vi "EMTS_Simulator_2017_V1_Tansmitter_One_Plane_Multi_Orientation_KF_Test_CV-RobertTest.vi"() -> ()   [LabVIEW 2014]
uses:
  <vilib>/Utility/error.llb/DialogType.ctl
  <vilib>/Utility/file.llb/Write To Spreadsheet File (DBL).vi
  <vilib>/measure/NI_MAPro.lvlib
panel:
  out "Times":i32
  out "U_norm":dbl[](array[numeric])
  out "Time needed (s)":dbl format="%.2f"
  out "Signal Frequency":dbl=1000.0 format="%.2f"
  out "Numeric":i32=49
  in  "DC  (V)":dbl=1.0 format="%_3f"
  in  "Ramp Voltage (V)":dbl=1.0 format="%_3f"
  out "concatenated string":string="100*a*t"
  in  "Reset Signal":bool=TRUE
  in  "Sampling info (sine)":cluster{"Fs":dbl, "#s":dbl}={"Fs"=100000.0, "#s"=1001.0} {"Fs" format="%.2p"}
  in  "Sampling info (DC)":cluster{"Fs":dbl, "#s":dbl}={"Fs"=100000.0, "#s"=1000.0} {"Fs" format="%.2p"}
  in  "Theta_Guess":dbl=90.0
  in  "Phi_Guess":dbl=90.0
  in  "Z_Guess":dbl=0.05
  in  "Y_Guess":dbl
  in  "X_Guess":dbl
  out "Measured Voltage":dbl[][](graph)
  in  "Noise On ?":bool=TRUE
  out "delta_t":dbl=0.01001
  out "#s":dbl=1001.0
  in  "Select Waveform":u16(ring) items=["Sine Wave", "Ramp Wave", "DC Wave"]
  in  "Sampling info (ramp)":cluster{"Fs":dbl, "#s":dbl}={"Fs"=100000.0, "#s"=1000.0} {"Fs" format="%.2p"}
  in  "Sine Frequency (Hz)":dbl=1000.0 format="%.2f"
  in  "Sine Voltage (V)":dbl=1.0 format="%0.2p"
  out "Signal Generation":waveform(dbl)(graph)={"t0"=timestamp(0 s since 1904-01-01), "dt"=1e-05, "Y"=array[1001 elements]}
  in  "Noise Level (dBW)":dbl=-80.0
  in  "Sensor static ?":bool=TRUE
  in  "Reference length":sgl=4.0
  in  "Yaw 1 (deg)  4":dbl=90.0
  in  "Pitch 1 (deg) 4":dbl
  in  "Roll 1 (deg) 4":dbl
  in  "Yaw 1 (deg)  3":dbl
  in  "Pitch 1 (deg) 3":dbl
  in  "Roll 1 (deg) 3":dbl
  in  "Yaw 1 (deg)  2":dbl=90.0
  in  "Pitch 1 (deg) 2":dbl=90.0
  in  "Roll 1 (deg) 2":dbl
  in  "Reference Point":cluster{"X (m)":sgl, "Y (m)":sgl, "Z (m)":sgl}
  out "Real Yaw 8":dbl
  out "Real Pitch 8":dbl=90.0
  out "Real Yaw 7":dbl=5.0
  out "Real Pitch 7":dbl
  out "Real Yaw 6":dbl=240.0
  out "Real Pitch6":dbl=30.0
  out "Real Yaw 5":dbl=120.0
  out "Real Pitch 5":dbl=100.0
  out "Real Yaw 4":dbl=120.0
  out "Real Pitch 4":dbl=60.0
  out "Real Yaw 3":dbl=90.0
  out "Real Pitch 3":dbl=30.0
  out "Real Yaw 2":dbl=33.0
  out "Real Pitch 2":dbl=63.0
  out "Real Yaw 1":dbl=-85.0
  out "Real Pitch 1":dbl=92.0
  out "XYZ Coil8":cluster{dbl, dbl, dbl}={-0.04600000008940697, 0.0, 0.0}
  out "XYZ Coil7":cluster{dbl, dbl, dbl}={0.05000000074505806, 0.009999999776482582, 0.0}
  out "XYZ Coil6":cluster{dbl, dbl, dbl}={0.05000000074505806, 0.10000000149011612, 0.0}
  out "XYZ Coil5":cluster{dbl, dbl, dbl}={0.1550000011920929, 0.0, 0.0}
  out "XYZ Coil4":cluster{dbl, dbl, dbl}={0.05000000074505806, -0.10000000149011612, 0.0010000000474974513}
  out "XYZ Coil3":cluster{dbl, dbl, dbl}={-0.05000000074505806, -0.10000000149011612, 0.0}
  out "XYZ Coil2":cluster{dbl, dbl, dbl}={-0.14800000190734863, 0.003000000026077032, -0.0010000000474974513}
  out "XYZ Coil1":cluster{dbl, dbl, dbl}={-0.049000002443790436, 0.10500000417232513, -0.0020000000949949026}
  in  "DYaw8":dbl
  in  "DPitch8":dbl
  in  "DZ8":sgl
  in  "DY8":sgl
  in  "DX8":sgl=0.004
  in  "DYaw7":dbl=5.0
  in  "DPitch7":dbl
  in  "DZ7":sgl
  in  "DY7":sgl=0.01
  in  "DX7":sgl
  in  "DYaw6":dbl
  in  "DPitch6":dbl
  in  "DZ6":sgl
  in  "DY6":sgl
  in  "DX6":sgl
  in  "DYaw5":dbl
  in  "DPitch5":dbl=10.0
  in  "DZ5":sgl
  in  "DY5":sgl
  in  "DX5":sgl=0.005
  in  "DYaw4":dbl
  in  "DPitch4":dbl
  in  "DZ4":sgl=0.001
  in  "DY4":sgl
  in  "DX4":sgl
  in  "DYaw3":dbl
  in  "DPitch3":dbl
  in  "DZ3":sgl
  in  "DY3":sgl
  in  "DX3":sgl
  in  "DYaw2":dbl=3.0
  in  "DPitch2":dbl=3.0
  in  "DZ2":sgl=-0.001
  in  "DY2":sgl=0.003
  in  "DX2":sgl=0.002
  in  "DYaw1":dbl=5.0
  in  "DPitch1":dbl=2.0
  in  "DZ1":sgl=-0.002
  in  "DY1":sgl=0.005
  in  "DX1":sgl=0.001
  out "Yaw (deg)":dbl=45.0
  out "Pitch (deg)":dbl=45.0
  out "Sensor coil move":cluster{"X (m)":sgl, "Y (m)":sgl, "Z (m)":sgl}={"X (m)"=0.0, "Y (m)"=0.0, "Z (m)"=0.12}
  in  "stop":bool
  in  "Transmitters accurate ?":bool=TRUE
  out "Real sensor's P&O":dbl[](array[numeric])=[-0.25, -0.25, 0.05000000074505806, -180.0, -180.0] format="%_6g"
  out "Simulated voltage induced by each transmitter coil (V)":dbl[](array[numeric])=[-0.021471154535231914, -0.017236602261565384, -0.01016434944143931, -0.0024446696112596913, 0.011573940229747934, 0.026417718734482783, 0.025183921853267847, 0.015931276239022865]
  out "Estimated sensor's P&O":dbl[](array[numeric])=[-0.10001654341217367, -0.09996105359602137, 0.0500756336809607, -0.007269984859161761, 90.04621343342399] format="%.4f"
  in  "Radius of the sensor coil (m)":dbl=0.0002832
  in  "Radius of the transmitter coils (m)":dbl=0.015
  in  "Turns of the sensor coil":dbl=500.0
  in  "Length of the transmitter coils (m)":dbl=0.03
  in  "Turns of the transmitter coils":dbl=207.0
  in  "Pitch (deg)":dbl=45.0
  in  "Yaw (deg)":dbl=45.0
  in  "Roll (deg)":dbl
  in  "Sensor coil":cluster{"X (m)":sgl, "Y (m)":sgl, "Z (m)":sgl}={"X (m)"=0.0, "Y (m)"=0.0, "Z (m)"=0.12}
  in  "Pitch 8 (deg)":dbl=90.0
  in  "Yaw 8 (deg)":dbl
  in  "Roll 8 (deg)":dbl
  in  "Coil 8":cluster{"X (m)":sgl, "Y (m)":sgl, "Z (m)":sgl}={"X (m)"=-0.05, "Y (m)"=0.0, "Z (m)"=0.0}
  in  "Pitch 7 (deg)":dbl
  in  "Yaw 7 (deg)":dbl
  in  "Roll 7 (deg)":dbl
  in  "Coil 7":cluster{"X (m)":sgl, "Y (m)":sgl, "Z (m)":sgl}={"X (m)"=0.05, "Y (m)"=0.0, "Z (m)"=0.0}
  in  "Pitch 6 (deg)":dbl=30.0
  in  "Yaw 6 (deg)":dbl=240.0
  in  "Roll 6 (deg)":dbl
  in  "Coil 6":cluster{"X (m)":sgl, "Y (m)":sgl, "Z (m)":sgl}={"X (m)"=0.05, "Y (m)"=0.1, "Z (m)"=0.0}
  in  "Pitch 5 (deg)":dbl=90.0
  in  "Yaw 5 (deg)":dbl=120.0
  in  "Roll 5 (deg)":dbl
  in  "Coil 5":cluster{"X (m)":sgl, "Y (m)":sgl, "Z (m)":sgl}={"X (m)"=0.15, "Y (m)"=0.0, "Z (m)"=0.0}
  in  "Pitch 4 (deg)":dbl=60.0
  in  "Yaw 4 (deg)":dbl=120.0
  in  "Roll 4 (deg)":dbl
  in  "Coil 4":cluster{"X (m)":sgl, "Y (m)":sgl, "Z (m)":sgl}={"X (m)"=0.05, "Y (m)"=-0.1, "Z (m)"=0.0}
  in  "Pitch 3 (deg)":dbl=30.0
  in  "Yaw 3 (deg)":dbl=90.0
  in  "Roll 3 (deg)":dbl
  in  "Coil 3":cluster{"X (m)":sgl, "Y (m)":sgl, "Z (m)":sgl}={"X (m)"=-0.05, "Y (m)"=-0.1, "Z (m)"=0.0}
  in  "Pitch 2 (deg)":dbl=60.0
  in  "Yaw 2 (deg)":dbl=30.0
  in  "Roll 2 (deg)":dbl
  in  "Coil 2":cluster{"X (m)":sgl, "Y (m)":sgl, "Z (m)":sgl}={"X (m)"=-0.15, "Y (m)"=0.0, "Z (m)"=0.0}
  in  "Coil 1":cluster{"X (m)":sgl, "Y (m)":sgl, "Z (m)":sgl}={"X (m)"=-0.05, "Y (m)"=0.1, "Z (m)"=0.0}
  in  "Pitch (deg)":dbl=90.0
  in  "Roll 1 (deg)":dbl
  in  "Yaw 1 (deg)":dbl=-90.0
  out "3D Picture":refnum<vi>(3d-picture)
  in  "path to JPEG file":path
  # "Simulation Tool for 8 Channel AC Electromagnetic tracking system developed in OvG University \n                                                                    Copy Right 2016 received @ OvGU"
  # "Manual control of transmitter coils' shift"
  # "Changing positions (m) and orientations (degree) of the transmitter coils"
  # "Set coil parameter"
  # "Set P&Os of transmitter coil array"
  # "Author: Mengfei Li\n mengfei.li@ovgu.de"
  # "X (m)"
  # "Y (m)"
  # "Set sensor's P&O"
  # "Z (m)"
  # "Phi (deg)"
  # "Theta (deg)"
  # "Real position and orientation of the transmitter coils"
  # "Signal Generation Panel"
  # "Visualization of transmitter coil array and sensor coil"
  # "Real positions (m) and orientations (degree) of the transmitter coils"
  # "Initial guess value for \nsensor pose estimation"
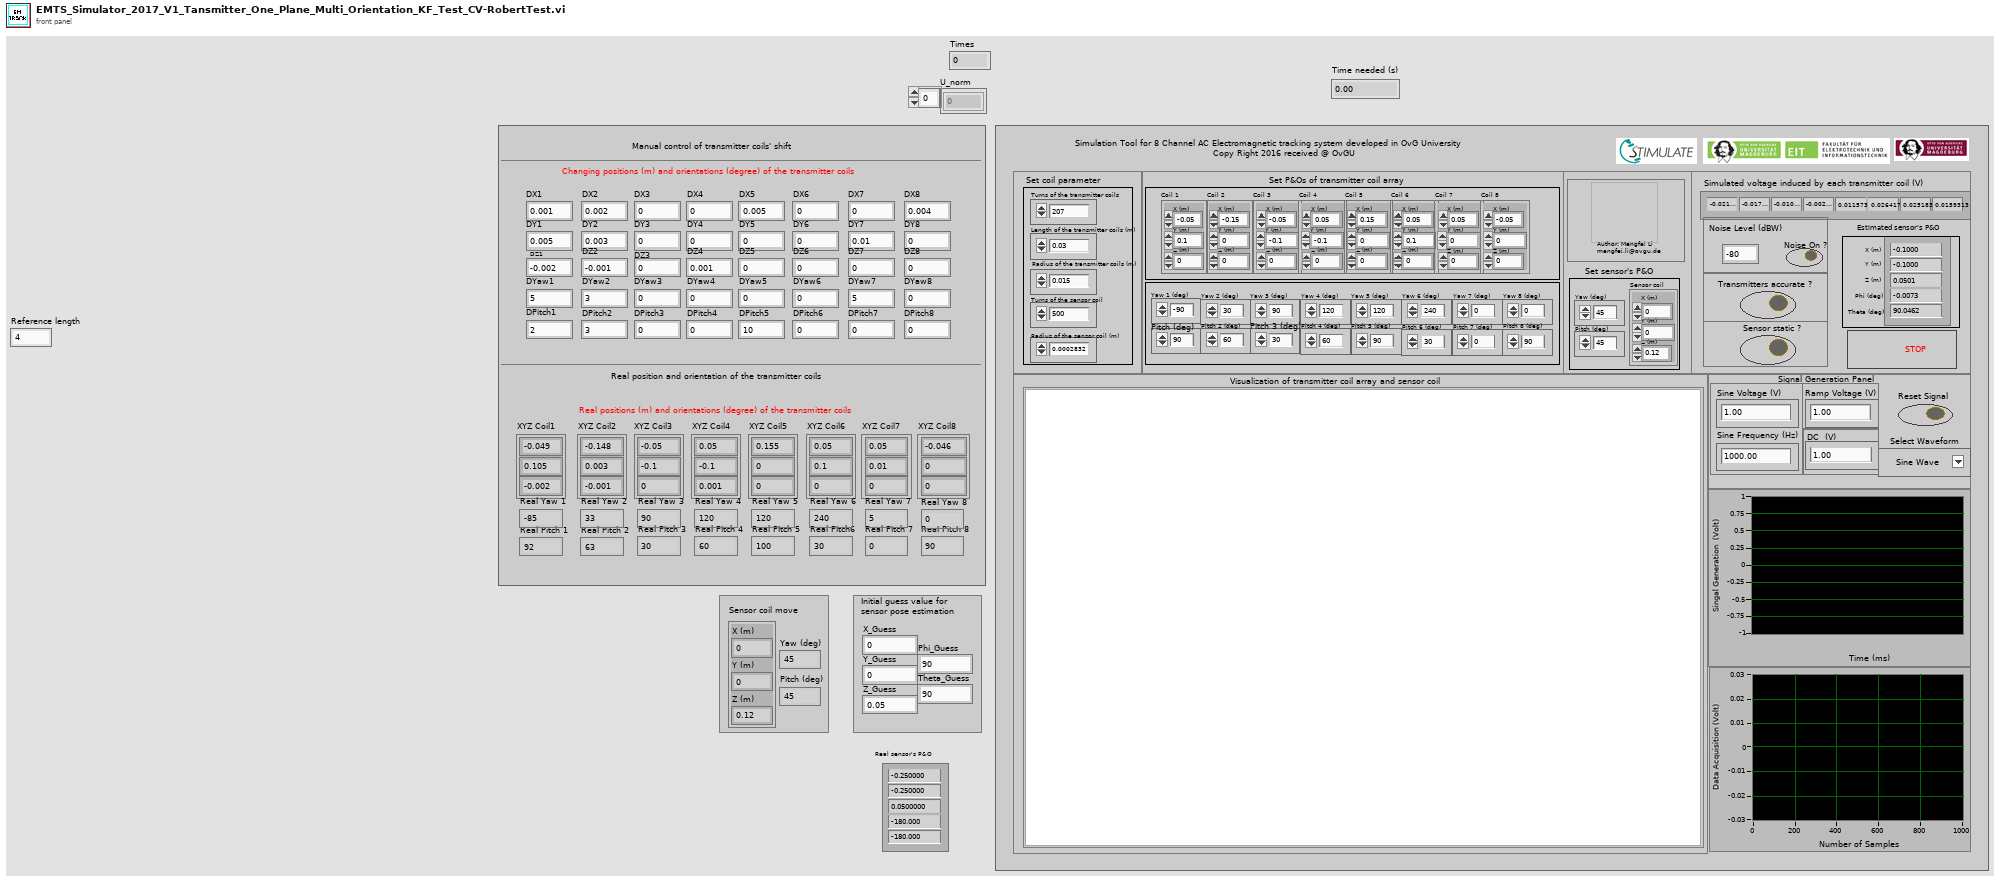
[diagram p1: front panel]
types:
  T1 = typedef "DialogType.ctl" = u16
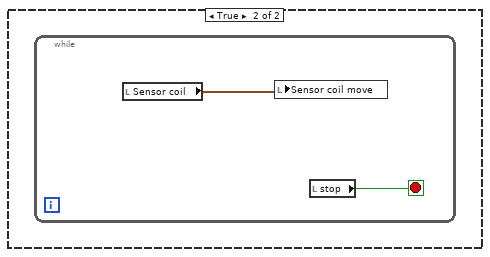
[diagram p2: hidden frame]
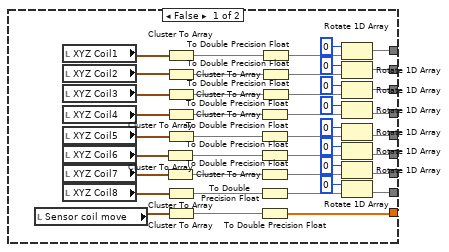
[diagram p4: hidden frame]
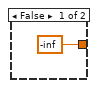
[diagram p5: hidden frame]
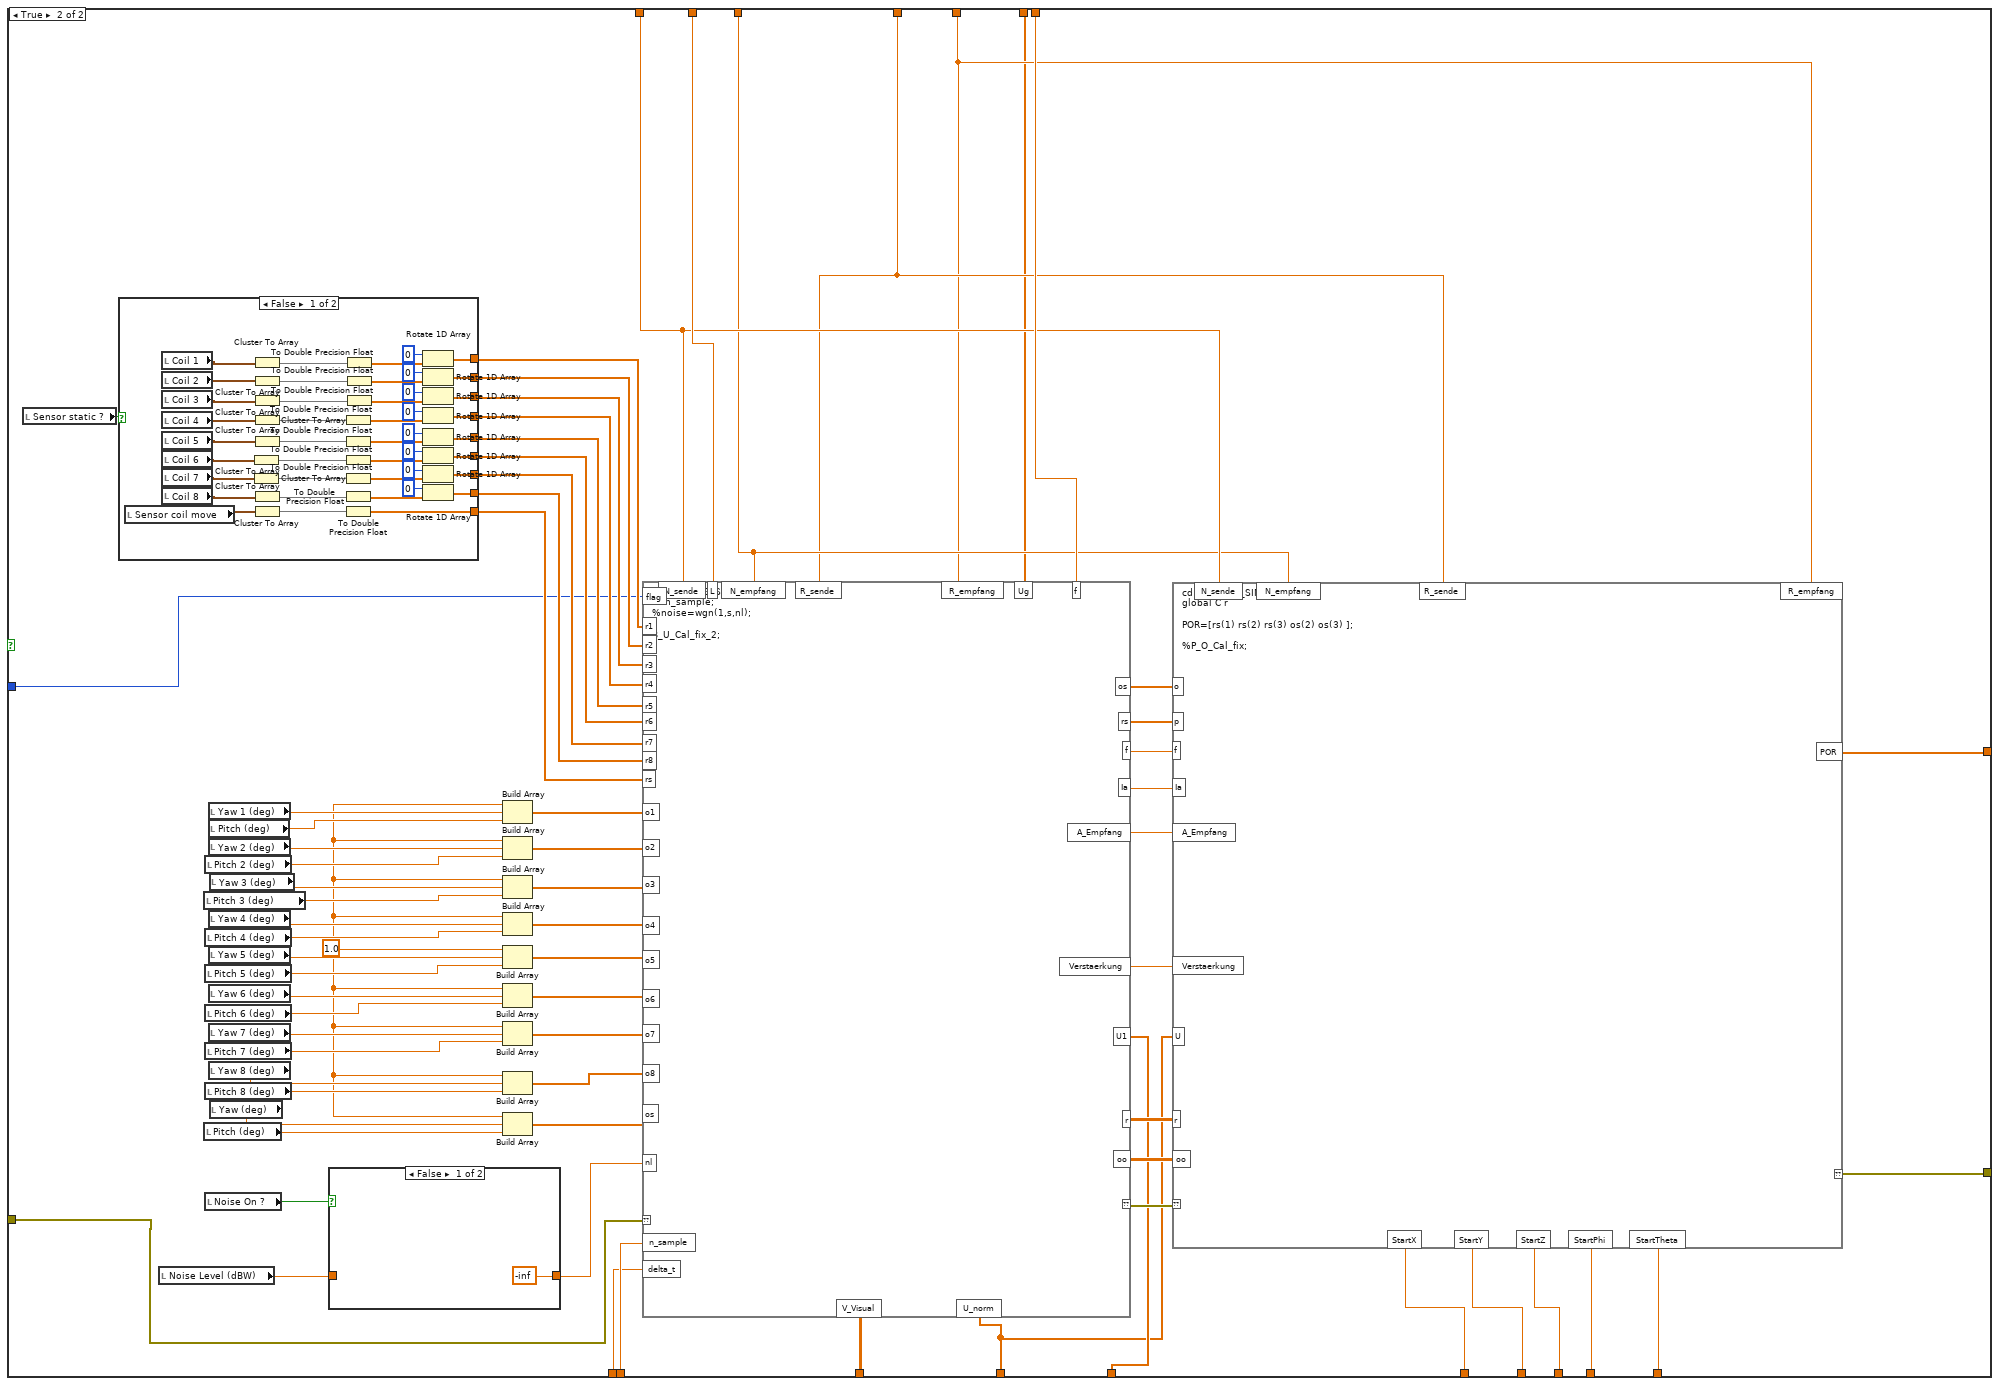
[diagram p6: hidden frame]
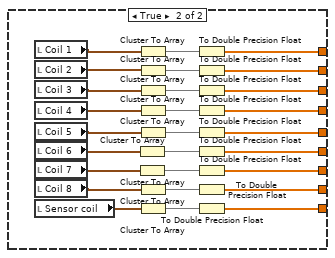
[diagram p7: hidden frame]
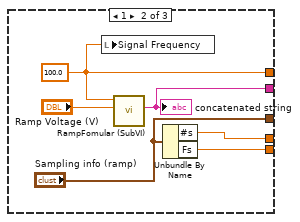
[diagram p12: hidden frame]
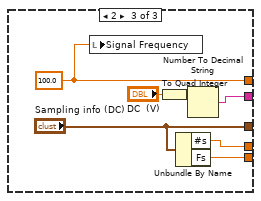
[diagram p13: hidden frame]
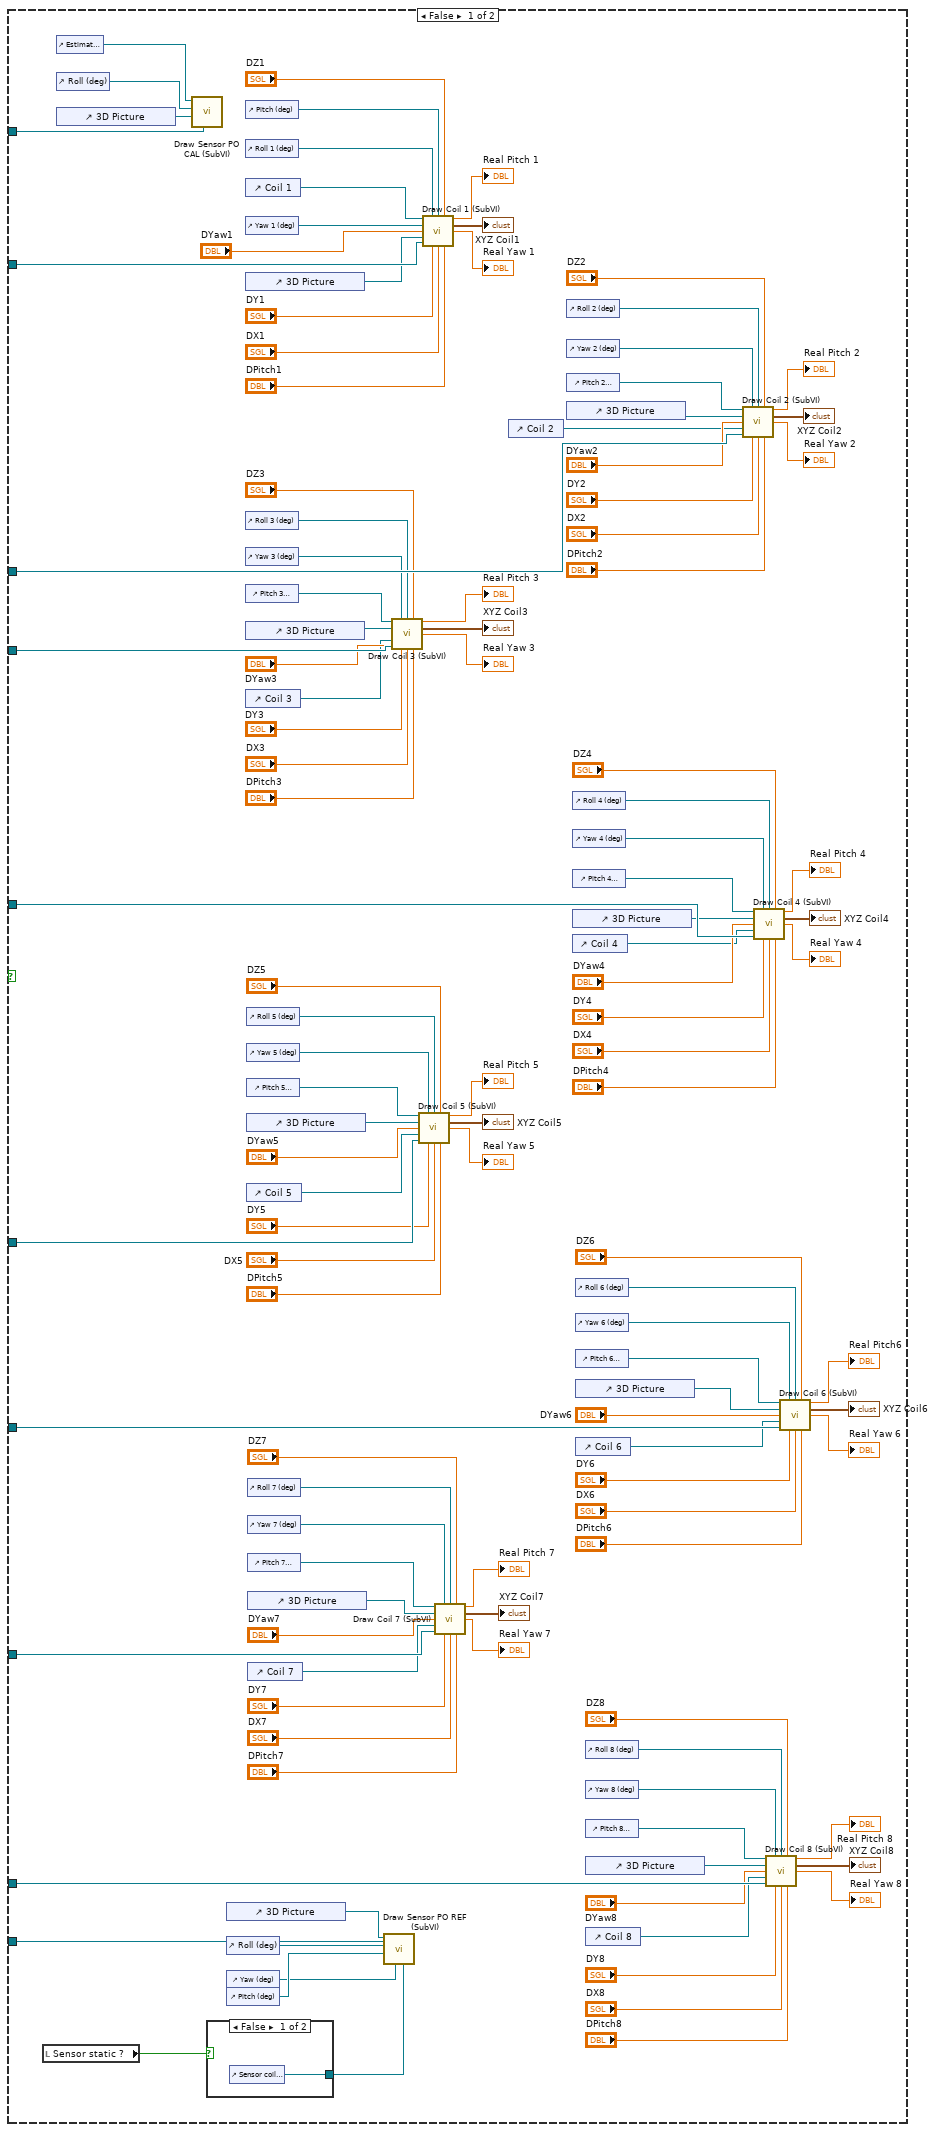
[diagram p14: hidden frame]
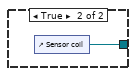
[diagram p15: hidden frame]
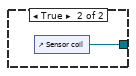
[diagram p16: hidden frame]
diagram:
  w7 = T1 3 items=["no dialog", "OK message", "continue or stop message", "OK message + warnings", "continue/stop + warnings"] ("type of dialog (OK msg:1)")
  # "This is an example here to move the sensor coil towards X, Y, Z axis. And this loop is where can be changed for testing the sensor movement models."
  # "Simulation of generated voltage"
  n1 = control-ref of="Length of the transmitter coils (m)"() -> (w15:refnum<vi>)
  n2 = control-ref of="Radius of the transmitter coils (m)"() -> (w16:refnum<vi>)
  n3 = call "Set Scenes (SubVI).vi"("Digital in"=w15, "path to JPEG file"="path to JPEG file", "reference"=w16) -> ("Scene:New Object"=w34:refnum<vi>, "Child 7"=w42:refnum<vi>, "SceneObject out"=w38:refnum<vi>, "Child"=w36:refnum<vi>, "Child 8"=w43:refnum<vi>, "Child 2"=w37:refnum<vi>, "Child 4"=w39:refnum<vi>, "Child 5"=w40:refnum<vi>, "Child 6"=w41:refnum<vi>)  [unwired: 4 in]
  n4 = control-ref of="Reference Point"() -> (w13:refnum<vi>)
  n5 = control-ref of="3D Picture"() -> (w14:refnum<vi>)
  n6 = while {
    stop <- w47 stop-if-true
    n7 = local read "Pitch (deg)"() -> (→"Pitch (deg)":dbl)
    n8 = local read "Yaw (deg)"() -> (→"Yaw (deg)":dbl)
    n9 = local read "stop"() -> (w47:bool)
    n10 = Wait (ms)(milliseconds to wait=u32 5) -> ()  [unwired: 1 out]
  }
  n11 = flat-sequence {
    tunnel: [w48] -> w5
    tunnel: w1 -> [w50]
    tunnel: w5 -> [w90]
    tunnel: [w89] -> w4
    frame #0 {
      n12 = Tick Count (ms)() -> (millisecond timer value=w48:u32)
      n13 = Wait (ms)(milliseconds to wait=u32 2000 ("millisecond timer value")) -> ()  [unwired: 1 out]
    }
    frame #1 {
      n14 = case shown="False" "Sensor static ?" {
        tunnel: w50 -> [w53 _]
        frame False {
          n15 = for {
            N: 100 -> [_]
            tunnel: w53 -> [w54]
            n16 = flat-sequence {
              tunnel: w54 -> [w72]
              frame #0 {
                n17 = local read "Sensor coil"() -> (w65:cluster{"X (m)":sgl, "Y (m)":sgl, "Z (m)":sgl})
                n18 = Unbundle(w65) -> ("X (m)"=w69:sgl, "Y (m)"=w56:sgl, "Z (m)"=w66:sgl)
                n19 = local read "Pitch (deg)"() -> (w59:dbl)
                n20 = Add(x=w69, y=sgl 0.001 ("x")) -> (x+y=w70:sgl)
                n21 = Add(x=sgl 0.0, y=w56) -> (x+y=w55:sgl)
                n22 = Add(x=sgl 0.0, y=w66) -> (x+y=w67:sgl)
                n23 = local read "Yaw (deg)"() -> (w62:dbl)
                n24 = Bundle(w70, w55, w67) -> (w64:cluster{sgl, sgl, sgl})  [unwired: 1 in]
                n25 = Add(x=w59, y=0.0) -> (x+y=w60:dbl)
                n26 = local write "Sensor coil move"(w64) -> ()
                n27 = local write "Sensor coil"(w64) -> ()
                n28 = local write "Pitch (deg)"(w60) -> ()
                n29 = Add(x=w62, y=0.0) -> (x+y=w61:dbl)
                n30 = local write "Yaw (deg)"(w61) -> ()
              }
              frame #1 {
                n31 = Set Occurrence(w72) -> ()
              }
              frame #2 {
                n32 = Wait (ms)(milliseconds to wait=u32 1200) -> ()  [unwired: 1 out]
              }
              frame #3 {
                n33 = local read "Simulated voltage induced by each transmitter coil (V)"() -> (w76:dbl[])
                n34 = local read "Real sensor's P&O"() -> (w74:dbl[])
                n35 = local read "U_norm"() -> (w75:dbl[])
                n36 = call-poly <vilib>:"Write To Spreadsheet File.vi"("format (%.3f)"="%.8f", "append to file? (new file:F)"=TRUE, "1D data"=w75, "file path (dialog if empty)"=path "d:/Um_Noise") -> ()  [unwired: 4 in, 1 out]
                n37 = call-poly <vilib>:"Write To Spreadsheet File.vi"("format (%.3f)"="%.8f", "append to file? (new file:F)"=TRUE, "1D data"=w74, "file path (dialog if empty)"=path "d:/POR") -> ()  [unwired: 4 in, 1 out]
                n38 = call-poly <vilib>:"Write To Spreadsheet File.vi"("format (%.3f)"="%.8f", "append to file? (new file:F)"=TRUE, "1D data"=w76, "file path (dialog if empty)"=path "d:/Um_NoNoise") -> ()  [unwired: 4 in, 1 out]
              }
              frame #4 {
                n39 = Wait (ms)(milliseconds to wait=u32 5) -> ()  [unwired: 1 out]
              }
            }
          }
        }
        frame True {
          n40 = while {
            stop <- w87 stop-if-true
            n41 = local read "Sensor coil"() -> (w88:cluster{"X (m)":sgl, "Y (m)":sgl, "Z (m)":sgl})
            n42 = local write "Sensor coil move"(w88) -> ()
            n43 = local read "stop"() -> (w87:bool)
          }
        }
      }
    }
    frame #2 {
      n44 = Tick Count (ms)() -> (millisecond timer value=w91:u32)
      n45 = Subtract(x=w91, y=w90) -> (x-y=w89:u32)
    }
  }
  n46 = call "Output Scenes (SubVI).vi"("SceneGraphDisplay in"=w14, "Yaw 1 (deg)  in"="Yaw 1 (deg)  2", "Roll 1 (deg) 3"="Roll 1 (deg) 3", "Roll 1 (deg) in"="Roll 1 (deg) 2", "Pitch 1 (deg) 3"="Pitch 1 (deg) 3", "Yaw 1 (deg)  4"="Yaw 1 (deg)  4", "Yaw 1 (deg)  3"="Yaw 1 (deg)  3", "Roll 1 (deg) 4"="Roll 1 (deg) 4", "Scene:New Object in"=w34, "Pitch 1 (deg) 4"="Pitch 1 (deg) 4", "reference"=w13, "Reference length"="Reference length", "Reference Point"="Reference Point", "Pitch 1 (deg) in"="Pitch 1 (deg) 2") -> ("SceneObject out"=w35:refnum<vi>, "Scene:New Object out"=w19:refnum<vi>, "Child"=w33:refnum<vi>)  [unwired: 3 in]
  n47 = while {
    tunnel: w43 -> [w103]
    tunnel: w42 -> [w104]
    tunnel: w41 -> [w102]
    tunnel: w40 -> [w101]
    tunnel: w39 -> [w100]
    tunnel: w38 -> [w99]
    tunnel: w37 -> [w98]
    tunnel: w36 -> [w97]
    tunnel: w35 -> [w96]
    tunnel: w33 -> [w95]
    tunnel: ["stop"] -> w30
    tunnel: w19 -> [w92]
    stop <- "stop" stop-if-true
    # "Loop 1: Coil Control and Visualization Loop"
    n48 = case shown="True" "Transmitters accurate ?" {
      tunnel: w104 -> [w227 w281]
      tunnel: w103 -> [w226 w280]
      tunnel: w102 -> [w225 w275]
      tunnel: w101 -> [w224 w270]
      tunnel: w100 -> [w223 w265]
      tunnel: w99 -> [w222 w260]
      tunnel: w98 -> [w221 w255]
      tunnel: w97 -> [w220 w250]
      tunnel: w96 -> [w219 w246]
      tunnel: w95 -> [w228 w245]
      frame False {
        n49 = local read "Sensor static ?"() -> (w107:bool)
        n50 = control-ref of="Estimated sensor's P&O"() -> (w177:refnum<vi>)
        n51 = control-ref of="Roll (deg)"() -> (w176:refnum<vi>)
        n52 = control-ref of="3D Picture"() -> (w175:refnum<vi>)
        n53 = call "Draw Sensor PO CAL (SubVI).vi"("Child"=w228, "SceneGraphDisp Refnum"=w175, "reference in"=w176, "Array in"=w177) -> ()  [unwired: 8 in]
        n54 = case shown="False" w107 {
          tunnel: [w229 w230] -> w106
          frame False {
            n55 = control-ref of="Sensor coil move"() -> (w229:refnum<vi>)
          }
          frame True {
            n56 = control-ref of="Sensor coil"() -> (w230:refnum<vi>)
          }
        }
        n57 = control-ref of="3D Picture"() -> (w108:refnum<vi>)
        n58 = control-ref of="Roll (deg)"() -> (w111:refnum<vi>)
        n59 = control-ref of="Yaw (deg)"() -> (w109:refnum<vi>)
        n60 = control-ref of="Pitch (deg)"() -> (w110:refnum<vi>)
        n61 = control-ref of="Pitch (deg)"() -> (w173:refnum<vi>)
        n62 = control-ref of="Roll 1 (deg)"() -> (w172:refnum<vi>)
        n63 = control-ref of="Coil 1"() -> (w174:refnum<vi>)
        n64 = control-ref of="Yaw 1 (deg)"() -> (w171:refnum<vi>)
        n65 = control-ref of="3D Picture"() -> (w170:refnum<vi>)
        n66 = control-ref of="Roll 3 (deg)"() -> (w158:refnum<vi>)
        n67 = control-ref of="Yaw 3 (deg)"() -> (w157:refnum<vi>)
        n68 = control-ref of="Pitch 3 (deg)"() -> (w159:refnum<vi>)
        n69 = control-ref of="3D Picture"() -> (w156:refnum<vi>)
        n70 = control-ref of="Coil 3"() -> (w155:refnum<vi>)
        n71 = control-ref of="Roll 5 (deg)"() -> (w142:refnum<vi>)
        n72 = control-ref of="Yaw 5 (deg)"() -> (w141:refnum<vi>)
        n73 = control-ref of="Pitch 5 (deg)"() -> (w143:refnum<vi>)
        n74 = control-ref of="3D Picture"() -> (w140:refnum<vi>)
        n75 = control-ref of="Coil 5"() -> (w139:refnum<vi>)
        n76 = control-ref of="Roll 7 (deg)"() -> (w126:refnum<vi>)
        n77 = control-ref of="Yaw 7 (deg)"() -> (w125:refnum<vi>)
        n78 = control-ref of="Pitch 7 (deg)"() -> (w127:refnum<vi>)
        n79 = control-ref of="3D Picture"() -> (w124:refnum<vi>)
        n80 = control-ref of="Coil 7"() -> (w123:refnum<vi>)
        n81 = call "Draw Sensor PO REF (SubVI).vi"("reference 4"=w106, "reference 3"=w109, "SceneObject in"=w219, "reference 2"=w110, "reference"=w111, "SceneGraphDisplay in"=w108) -> ()  [unwired: 6 in]
        n82 = call "Draw Coil 3 (SubVI).vi"("Digital in"=w159, "reference 3"=w157, "reference in"=w158, "DZ3"="DZ3", "SceneGraphDisp Refnum"=w156, "DPitch3"="DYaw3", "reference 4"=w155, "Child 6"=w225, "DY3"="DY3", "DX3"="DX3", "DYaw3"="DPitch3") -> ("Real Yaw 3"=→"Real Pitch 3":dbl, "XYZ Coil3"=→"XYZ Coil3":cluster{dbl, dbl, dbl}, "Real Pitch 3"=→"Real Yaw 3":dbl)  [unwired: 2 in]
        n83 = call "Draw Coil 5 (SubVI).vi"("Digital in"=w143, "reference 3"=w141, "reference in"=w142, "DZ5"="DZ5", "SceneGraphDisp Refnum"=w140, "DPitch5"="DYaw5", "reference 4"=w139, "Child 4"=w223, "DY5"="DY5", "DX5"="DX5", "DYaw5"="DPitch5") -> ("Real Yaw 5"=→"Real Pitch 5":dbl, "XYZ Coil5"=→"XYZ Coil5":cluster{dbl, dbl, dbl}, "Real Pitch 5"=→"Real Yaw 5":dbl)  [unwired: 2 in]
        n84 = call "Draw Coil 1 (SubVI).vi"("Cluster in"=w174, "reference 3"=w172, "reference in"=w173, "DZ1"="DZ1", "reference 4"=w171, "DPitch1"="DYaw1", "SceneGraphDisp Refnum"=w170, "Child 7"=w227, "DY1"="DY1", "DX1"="DX1", "DYaw1"="DPitch1") -> ("Real Yaw 1"=→"Real Pitch 1":dbl, "XYZ Coil1"=→"XYZ Coil1":cluster{dbl, dbl, dbl}, "Real Pitch 1"=→"Real Yaw 1":dbl)  [unwired: 2 in]
        n85 = call "Draw Coil 7 (SubVI).vi"("Digital in"=w127, "reference 3"=w125, "reference in"=w126, "DZ7"="DZ7", "SceneGraphDisp Refnum"=w124, "DPitch7"="DYaw7", "reference 4"=w123, "Child in"=w221, "DY7"="DY7", "DX7"="DX7", "DYaw7"="DPitch7") -> ("Real Yaw 7"=→"Real Pitch 7":dbl, "XYZ Coil7"=→"XYZ Coil7":cluster{dbl, dbl, dbl}, "Real Pitch 7"=→"Real Yaw 7":dbl)  [unwired: 2 in]
        n86 = control-ref of="Coil 2"() -> (w162:refnum<vi>)
        n87 = control-ref of="Roll 2 (deg)"() -> (w165:refnum<vi>)
        n88 = control-ref of="Yaw 2 (deg)"() -> (w164:refnum<vi>)
        n89 = control-ref of="Pitch 2 (deg)"() -> (w166:refnum<vi>)
        n90 = control-ref of="3D Picture"() -> (w163:refnum<vi>)
        n91 = control-ref of="Roll 4 (deg)"() -> (w150:refnum<vi>)
        n92 = control-ref of="Yaw 4 (deg)"() -> (w149:refnum<vi>)
        n93 = control-ref of="Pitch 4 (deg)"() -> (w151:refnum<vi>)
        n94 = control-ref of="3D Picture"() -> (w148:refnum<vi>)
        n95 = control-ref of="Coil 4"() -> (w147:refnum<vi>)
        n96 = control-ref of="Roll 6 (deg)"() -> (w134:refnum<vi>)
        n97 = control-ref of="Yaw 6 (deg)"() -> (w133:refnum<vi>)
        n98 = control-ref of="Pitch 6 (deg)"() -> (w135:refnum<vi>)
        n99 = control-ref of="3D Picture"() -> (w132:refnum<vi>)
        n100 = control-ref of="Coil 6"() -> (w131:refnum<vi>)
        n101 = control-ref of="Roll 8 (deg)"() -> (w118:refnum<vi>)
        n102 = control-ref of="Yaw 8 (deg)"() -> (w117:refnum<vi>)
        n103 = control-ref of="Pitch 8 (deg)"() -> (w119:refnum<vi>)
        n104 = control-ref of="3D Picture"() -> (w116:refnum<vi>)
        n105 = control-ref of="Coil 8"() -> (w115:refnum<vi>)
        n106 = call "Draw Coil 2 (SubVI).vi"("Digital in"=w166, "reference 3"=w164, "reference in"=w165, "DZ2"="DZ2", "SceneGraphDisp Refnum"=w163, "DPitch2"="DYaw2", "reference 4"=w162, "Child 8"=w226, "DY2"="DY2", "DX2"="DX2", "DYaw2"="DPitch2") -> ("Real Yaw 2"=→"Real Pitch 2":dbl, "XYZ Coil2"=→"XYZ Coil2":cluster{dbl, dbl, dbl}, "Numeric"=→"Real Yaw 2":dbl)  [unwired: 2 in]
        n107 = call "Draw Coil 4 (SubVI).vi"("Digital in"=w151, "reference 3"=w149, "reference in"=w150, "DZ4"="DZ4", "SceneGraphDisp Refnum"=w148, "DPitch4"="DYaw4", "reference 4"=w147, "Child 5"=w224, "DY4"="DY4", "DX4"="DX4", "DYaw4"="DPitch4") -> ("Real Yaw 4"=→"Real Pitch 4":dbl, "XYZ Coil4"=→"XYZ Coil4":cluster{dbl, dbl, dbl}, "Real Pitch 4"=→"Real Yaw 4":dbl)  [unwired: 2 in]
        n108 = call "Draw Coil 8 (SubVI).vi"("Digital in"=w119, "reference 3"=w117, "reference in"=w118, "DZ8"="DZ8", "SceneGraphDisp Refnum"=w116, "DPitch8"="DYaw8", "reference 4"=w115, "Child"=w220, "DY8"="DY8", "DX8"="DX8", "DYaw8"="DPitch8") -> ("Real Yaw 8"=→"Real Pitch 8":dbl, "XYZ Coil8"=→"XYZ Coil8":cluster{dbl, dbl, dbl}, "Real Pitch 8"=→"Real Yaw 8":dbl)  [unwired: 2 in]
        n109 = call "Draw Coil 6 (SubVI).vi"("Digital in"=w135, "reference 3"=w133, "reference in"=w134, "DZ6"="DZ6", "SceneGraphDisp Refnum"=w132, "DPitch6"="DYaw6", "reference 4"=w131, "SceneObject in"=w222, "DY6"="DY6", "DX6"="DX6", "DYaw6"="DPitch6") -> ("Real Yaw 6"=→"Real Pitch6":dbl, "XYZ Coil6"=→"XYZ Coil6":cluster{dbl, dbl, dbl}, "Real Pitch 6"=→"Real Yaw 6":dbl)  [unwired: 2 in]
      }
      frame True {
        n110 = control-ref of="3D Picture"() -> (w240:refnum<vi>)
        n111 = control-ref of="3D Picture"() -> (w238:refnum<vi>)
        n112 = control-ref of="3D Picture"() -> (w244:refnum<vi>)
        n113 = control-ref of="Estimated sensor's P&O"() -> (w243:refnum<vi>)
        n114 = control-ref of="Roll (deg)"() -> (w242:refnum<vi>)
        n115 = control-ref of="3D Picture"() -> (w236:refnum<vi>)
        n116 = control-ref of="3D Picture"() -> (w234:refnum<vi>)
        n117 = local read "Sensor static ?"() -> (w232:bool)
        n118 = call "Draw Coil 2_1 (SubVI).vi"("Roll 2 (deg)"="Roll 2 (deg)", "Yaw 2 (deg)"="Pitch 2 (deg)", "Pitch 2 (deg)"="Yaw 2 (deg)", "Child 8"=w280, "Coil in"="Coil 2", "SceneGraphDisplay in"=w240) -> ()  [unwired: 6 in]
        n119 = call "Draw Sensor PO CAL_1 (SubVI).vi"("Child"=w245, "reference 2"=w242, "reference"=w243, "SceneGraphDisplay in"=w244) -> ()  [unwired: 8 in]
        n120 = call "Draw Coil 4_1 (SubVI).vi"("Roll 4 (deg)"="Roll 4 (deg)", "Yaw 4 (deg)"="Pitch 4 (deg)", "Pitch 4 (deg)"="Yaw 4 (deg)", "SceneGraphDisp Refnum"=w238, "Coil 4"="Coil 4", "SceneObject in"=w270) -> ()  [unwired: 6 in]
        n121 = call "Draw Coil 6_1 (SubVI).vi"("Roll 6 (deg)"="Roll 6 (deg)", "Yaw 6 (deg)"="Pitch 6 (deg)", "Pitch 6 (deg)"="Yaw 6 (deg)", "SceneObject in"=w260, "Coil 6"="Coil 6", "SceneGraphDisplay in"=w236) -> ()  [unwired: 6 in]
        n122 = call "Draw Coil 8_1 (SubVI).vi"("Roll 8 (deg)"="Roll 8 (deg)", "Yaw 8 (deg)"="Pitch 8 (deg)", "Pitch 8 (deg)"="Yaw 8 (deg)", "Child"=w250, "Coil 8"="Coil 8", "SceneGraphDisplay in"=w234) -> ()  [unwired: 6 in]
        n123 = case shown="False" w232 {
          tunnel: [w290 w291] -> w231
          frame False {
            n124 = control-ref of="Sensor coil move"() -> (w290:refnum<vi>)
          }
          frame True {
            n125 = control-ref of="Sensor coil"() -> (w291:refnum<vi>)
          }
        }
        n126 = control-ref of="3D Picture"() -> (w237:refnum<vi>)
        n127 = control-ref of="3D Picture"() -> (w233:refnum<vi>)
        n128 = control-ref of="3D Picture"() -> (w235:refnum<vi>)
        n129 = control-ref of="3D Picture"() -> (w239:refnum<vi>)
        n130 = control-ref of="3D Picture"() -> (w241:refnum<vi>)
        n131 = call "Draw Coil 5_1 (SubVI).vi"("Roll 5 (deg)"="Roll 5 (deg)", "Yaw 5 (deg)"="Pitch 5 (deg)", "Pitch 5 (deg)"="Yaw 5 (deg)", "Child 4"=w265, "Coil 5"="Coil 5", "SceneGraphDisplay in"=w237) -> ()  [unwired: 6 in]
        n132 = call "Draw Coil 7_1 (SubVI).vi"("Roll 7 (deg)"="Roll 7 (deg)", "Yaw 7 (deg)"="Pitch 7 (deg)", "Pitch 7 (deg)"="Yaw 7 (deg)", "Child in"=w255, "Coil 7"="Coil 7", "SceneGraphDisplay in"=w235) -> ()  [unwired: 6 in]
        n133 = call "Draw Coil 3_1 (SubVI).vi"("Roll 3 (deg)"="Roll 3 (deg)", "Yaw 3 (deg)"="Pitch 3 (deg)", "Pitch 3 (deg)"="Yaw 3 (deg)", "SceneGraphDisp Refnum"=w239, "Coil 3"="Coil 3", "SceneObject in"=w275) -> ()  [unwired: 6 in]
        n134 = call "Draw Sensor PO REF_1 (SubVI).vi"("Roll (deg)"="Roll (deg)", "SceneObject in"=w246, "Pitch (deg)"="Yaw (deg)", "reference"=w231, "Yaw (deg)"="Pitch (deg)", "SceneGraphDisplay in"=w233) -> ()  [unwired: 6 in]
        n135 = call "Draw Coil 1_1 (SubVI).vi"("Roll 1 (deg)"="Roll 1 (deg)", "Yaw 1 (deg)"="Pitch (deg)", "Pitch 1 (deg)"="Yaw 1 (deg)", "Child 7"=w281, "Coil 1"="Coil 1", "SceneGraphDisplay in"=w241) -> ()  [unwired: 6 in]
      }
    }
    n136 = Wait (ms)(milliseconds to wait=u32 20) -> ()  [unwired: 1 out]
    "3D Picture" <- w92
  }
  n137 = local read "stop"() -> (w32:bool)
  n138 = Not Or(1:w32, 2:w30) -> (0:w31:bool)
  n139 = local write "stop"(w31) -> ()
  n140 = disable-structure shown="Disabled" {
    frame Disabled {
      n141 = flat-sequence {
        frame #0 {
          n142 = Wait (ms)(milliseconds to wait=u32 4000) -> ()  [unwired: 1 out]
        }
        frame #1 {
          n143 = for {
            N: 50 -> [_]
            shift-right: [w302] -> _
            shift-left: _ -> [_]
            shift-right: [w301] -> _
            shift-left: _ -> [w300]
            shift-left: _ -> [w294]
            shift-left: _ -> [w296]
            i -> [w305]
            n144 = Not Equal?(x=w300, y=w294) -> (x != y?=w299:bool[])
            n145 = Index Array(array=w299, index=0) -> (element=w297:bool)
            n146 = case shown="False" w297 {
              tunnel: [i32[] [0, 0, 0, 0, 0] w312] -> w295
              tunnel: w294 -> [_ w312]
              frame False {
              }
              frame True {
              }
            }
            n147 = Wait (ms)(milliseconds to wait=u32 500) -> ()  [unwired: 1 out]
            n148 = call-poly <vilib>:"Write To Spreadsheet File.vi"("format (%.3f)"="%.8f", "append to file? (new file:F)"=TRUE, "1D data"=w296, "file path (dialog if empty)"=path "d:/test2016/paper2/eval1/POE") -> ()  [unwired: 4 in, 1 out]
            n149 = local read "Estimated sensor's P&O"() -> (w302:dbl[])
            n150 = local read "Real sensor's P&O"() -> (w301:dbl[])
            n151 = call-poly <vilib>:"Write To Spreadsheet File.vi"("format (%.3f)"="%.8f", "append to file? (new file:F)"=TRUE, "1D data"=w295, "file path (dialog if empty)"=path "d:/test2016/paper2/eval1/POR") -> ()  [unwired: 4 in, 1 out]
            "Numeric" <- w305
          }
        }
      }
    }
    frame Enabled {
    }
  }
  n152 = Generate Occurrence() -> (w1:refnum<k4>)
  n153 = while {
    tunnel: [w319] -> w6
    tunnel: "X_Guess" -> [w318]
    tunnel: "Y_Guess" -> [w317]
    tunnel: "Z_Guess" -> [w316]
    tunnel: "Phi_Guess" -> [w315]
    tunnel: "Theta_Guess" -> [w314]
    tunnel: w1 -> [w313]
    stop <- w320 stop-if-true
    n154 = flat-sequence {
      tunnel: w313 -> [w321]
      tunnel: [w344] -> w320
      tunnel: [w336] -> w319
      tunnel: w318 -> [w327]
      tunnel: w317 -> [w326]
      tunnel: w316 -> [w325]
      tunnel: w315 -> [w324]
      tunnel: w314 -> [w323]
      frame #0 {
        n155 = Wait on Occurrence(2:w321) -> ()  [unwired: 2 in, 1 out]
      }
      frame #1 {
        n156 = local read "Transmitters accurate ?"() -> (w337:bool)
        n157 = local read "Select Waveform"() -> (w331:u16)
        n158 = local read "Signal Generation"() -> (w330:waveform(dbl))
        n159 = Unbundle By Name(w330) -> ("Y"=w329:dbl[])
        n160 = local read "#s"() -> (w333:dbl)
        n161 = local read "delta_t"() -> (w332:dbl)
        n162 = local read "Sine Frequency (Hz)"() -> (w334:dbl)
        n163 = case shown="False" w337 {
          tunnel: w334 -> [w422 w564]
          tunnel: "Length of the transmitter coils (m)" -> [w423 w563]
          tunnel: "Turns of the transmitter coils" -> [w419 w559]
          tunnel: "Turns of the sensor coil" -> [w418 w558]
          tunnel: "Radius of the transmitter coils (m)" -> [w417 w557]
          tunnel: "Radius of the sensor coil (m)" -> [w416 w556]
          tunnel: [w420 w533] -> w345
          tunnel: [w421 w551] -> w343
          tunnel: [w390 w548] -> w336
          tunnel: errorcluster {"status"=FALSE, "code"=0, "source"=""} ("error in") -> [w385 w532]
          tunnel: w333 -> [w389 w547]
          tunnel: w332 -> [w388 w546]
          tunnel: w331 -> [w387 w545]
          tunnel: w329 -> [w386 w544]
          tunnel: [w381 w540] -> w328
          tunnel: w327 -> [w379 w534]
          tunnel: w326 -> [w378 w539]
          tunnel: w325 -> [w377 w538]
          tunnel: w324 -> [w376 w537]
          tunnel: w323 -> [w375 w536]
          tunnel: [w347 w531] -> w322
          frame False {
            w374 = 1.0
            w442 = 1.0
            n164 = local read "Sensor static ?"() -> (w348:bool)
            n165 = case shown="True" w348 {
              tunnel: [w467 w508] -> w430
              tunnel: [w459 w516] -> w415
              tunnel: [w460 w515] -> w414
              tunnel: [w461 w514] -> w413
              tunnel: [w462 w513] -> w412
              tunnel: [w463 w512] -> w411
              tunnel: [w464 w511] -> w410
              tunnel: [w465 w510] -> w409
              tunnel: [w466 w509] -> w408
              frame False {
                n166 = local read "Sensor coil move"() -> (w468:cluster{"X (m)":sgl, "Y (m)":sgl, "Z (m)":sgl})
                n167 = local read "XYZ Coil1"() -> (w501:cluster{dbl, dbl, dbl})
                n168 = local read "XYZ Coil2"() -> (w500:cluster{dbl, dbl, dbl})
                n169 = local read "XYZ Coil3"() -> (w499:cluster{dbl, dbl, dbl})
                n170 = local read "XYZ Coil4"() -> (w498:cluster{dbl, dbl, dbl})
                n171 = local read "XYZ Coil5"() -> (w497:cluster{dbl, dbl, dbl})
                n172 = local read "XYZ Coil6"() -> (w496:cluster{dbl, dbl, dbl})
                n173 = local read "XYZ Coil7"() -> (w495:cluster{dbl, dbl, dbl})
                n174 = local read "XYZ Coil8"() -> (w494:cluster{dbl, dbl, dbl})
                n175 = Cluster To Array(cluster=w496) -> (array=w489:dbl[])
                n176 = Cluster To Array(cluster=w495) -> (array=w488:dbl[])
                n177 = Cluster To Array(cluster=w501) -> (array=w477:dbl[])
                n178 = Cluster To Array(cluster=w500) -> (array=w493:dbl[])
                n179 = Cluster To Array(cluster=w499) -> (array=w492:dbl[])
                n180 = Cluster To Array(cluster=w498) -> (array=w491:dbl[])
                n181 = Cluster To Array(cluster=w497) -> (array=w490:dbl[])
                n182 = Cluster To Array(cluster=w494) -> (array=w487:dbl[])
                n183 = Cluster To Array(cluster=w468) -> (array=w486:sgl[])
                n184 = To Double Precision Float(number=w491) -> (double precision float=w482:dbl[])
                n185 = To Double Precision Float(number=w490) -> (double precision float=w481:dbl[])
                n186 = To Double Precision Float(number=w489) -> (double precision float=w480:dbl[])
                n187 = To Double Precision Float(number=w488) -> (double precision float=w479:dbl[])
                n188 = To Double Precision Float(number=w487) -> (double precision float=w478:dbl[])
                n189 = To Double Precision Float(number=w486) -> (double precision float=w467:dbl[])
                n190 = To Double Precision Float(number=w477) -> (double precision float=w485:dbl[])
                n191 = To Double Precision Float(number=w493) -> (double precision float=w484:dbl[])
                n192 = To Double Precision Float(number=w492) -> (double precision float=w483:dbl[])
                n193 = Rotate 1D Array(1:w485, 2:0 ("n")) -> (0:w459:dbl[])
                n194 = Rotate 1D Array(1:w484, 2:0 ("n")) -> (0:w460:dbl[])
                n195 = Rotate 1D Array(1:w483, 2:0 ("n")) -> (0:w461:dbl[])
                n196 = Rotate 1D Array(1:w482, 2:0 ("n")) -> (0:w462:dbl[])
                n197 = Rotate 1D Array(1:w481, 2:0 ("n")) -> (0:w463:dbl[])
                n198 = Rotate 1D Array(1:w480, 2:0 ("n")) -> (0:w464:dbl[])
                n199 = Rotate 1D Array(1:w479, 2:0 ("n")) -> (0:w465:dbl[])
                n200 = Rotate 1D Array(1:w478, 2:0 ("n")) -> (0:w466:dbl[])
              }
              frame True {
                n201 = local read "XYZ Coil1"() -> (w528:cluster{dbl, dbl, dbl})
                n202 = local read "XYZ Coil2"() -> (w527:cluster{dbl, dbl, dbl})
                n203 = local read "XYZ Coil3"() -> (w507:cluster{dbl, dbl, dbl})
                n204 = local read "XYZ Coil4"() -> (w506:cluster{dbl, dbl, dbl})
                n205 = local read "XYZ Coil5"() -> (w505:cluster{dbl, dbl, dbl})
                n206 = local read "XYZ Coil6"() -> (w504:cluster{dbl, dbl, dbl})
                n207 = local read "XYZ Coil7"() -> (w503:cluster{dbl, dbl, dbl})
                n208 = local read "XYZ Coil8"() -> (w502:cluster{dbl, dbl, dbl})
                n209 = local read "Sensor coil"() -> (w526:cluster{"X (m)":sgl, "Y (m)":sgl, "Z (m)":sgl})
                n210 = Cluster To Array(cluster=w504) -> (array=w521:dbl[])
                n211 = Cluster To Array(cluster=w503) -> (array=w520:dbl[])
                n212 = Cluster To Array(cluster=w528) -> (array=w517:dbl[])
                n213 = Cluster To Array(cluster=w527) -> (array=w525:dbl[])
                n214 = Cluster To Array(cluster=w507) -> (array=w524:dbl[])
                n215 = Cluster To Array(cluster=w506) -> (array=w523:dbl[])
                n216 = Cluster To Array(cluster=w505) -> (array=w522:dbl[])
                n217 = Cluster To Array(cluster=w502) -> (array=w519:dbl[])
                n218 = Cluster To Array(cluster=w526) -> (array=w518:sgl[])
                n219 = To Double Precision Float(number=w517) -> (double precision float=w516:dbl[])
                n220 = To Double Precision Float(number=w525) -> (double precision float=w515:dbl[])
                n221 = To Double Precision Float(number=w524) -> (double precision float=w514:dbl[])
                n222 = To Double Precision Float(number=w523) -> (double precision float=w513:dbl[])
                n223 = To Double Precision Float(number=w522) -> (double precision float=w512:dbl[])
                n224 = To Double Precision Float(number=w521) -> (double precision float=w511:dbl[])
                n225 = To Double Precision Float(number=w520) -> (double precision float=w510:dbl[])
                n226 = To Double Precision Float(number=w519) -> (double precision float=w509:dbl[])
                n227 = To Double Precision Float(number=w518) -> (double precision float=w508:dbl[])
              }
            }
            n228 = local read "Real Pitch 1"() -> (w457:dbl)
            n229 = local read "Real Pitch 2"() -> (w455:dbl)
            n230 = local read "Real Pitch 3"() -> (w453:dbl)
            n231 = local read "Real Pitch 4"() -> (w451:dbl)
            n232 = local read "Real Pitch 5"() -> (w449:dbl)
            n233 = local read "Real Pitch 7"() -> (w445:dbl)
            n234 = local read "Real Pitch 8"() -> (w443:dbl)
            n235 = local read "Real Pitch6"() -> (w447:dbl)
            n236 = local read "Pitch (deg)"() -> (w441:dbl)
            n237 = local read "Yaw (deg)"() -> (w440:dbl)
            n238 = local read "Real Yaw 1"() -> (w458:dbl)
            n239 = local read "Real Yaw 2"() -> (w456:dbl)
            n240 = local read "Real Yaw 3"() -> (w454:dbl)
            n241 = local read "Real Yaw 4"() -> (w452:dbl)
            n242 = local read "Real Yaw 5"() -> (w450:dbl)
            n243 = local read "Real Yaw 6"() -> (w448:dbl)
            n244 = local read "Real Yaw 7"() -> (w446:dbl)
            n245 = local read "Real Yaw 8"() -> (w444:dbl)
            n246 = case shown="True" "Noise On ?" {
              tunnel: [-inf w530] -> w382
              tunnel: "Noise Level (dBW)" -> [_ w530]
              frame False {
              }
              frame True {
              }
            }
            n247 = Build Array(w442, w458, w457) -> (w439:dbl[])
            n248 = Build Array(w442, w456, w455) -> (w438:dbl[])
            n249 = Build Array(w442, w454, w453) -> (w437:dbl[])
            n250 = Build Array(w442, w452, w451) -> (w436:dbl[])
            n251 = Build Array(w442, w450, w449) -> (w435:dbl[])
            n252 = Build Array(w442, w448, w447) -> (w434:dbl[])
            n253 = Build Array(w442, w446, w445) -> (w433:dbl[])
            n254 = Build Array(w442, w444, w443) -> (w432:dbl[])
            n255 = Build Array(w442, w441, w440) -> (w431:dbl[])
            n256 = script code="cd ('C:\\EMTS_SIMU')\ns=n_sample;\n% noise=wgn(1,s,nl);\n\nB_U_Cal_fix_2;"("??"=w385, "r1"=w415, "r2"=w414, "r3"=w413, "r4"=w412, "r5"=w411, "r6"=w410, "r7"=w409, "r8"=w408, "rs"=w430, "o1"=w439, "o2"=w438, "o3"=w437, "o4"=w436, "o5"=w435, "o6"=w434, "o7"=w433, "o8"=w432, "os"=w431, "N_sende"=w419, "L"=w423, "N_empfang"=w418, "R_sende"=w417, "R_empfang"=w416, "Ug"=w386, "f"=w422, "nl"=w382, "n_sample"=w389, "delta_t"=w388, "flag"=w387) -> ("??"=w391:errorcluster, "rs"=w429:dbl[], "f"=w428:dbl, "os"=w427:dbl[], "Ia"=w426:dbl, "A_Empfang"=w425:dbl, "Verstaerkung"=w424:dbl, "U1"=w420:dbl[], "V_Visual"=w381:dbl[][], "U_norm"=w347:dbl[])
            n257 = local read "Pitch 3 (deg)"() -> (w363:dbl)
            n258 = local read "Pitch 2 (deg)"() -> (w361:dbl)
            n259 = local read "Pitch 4 (deg)"() -> (w365:dbl)
            n260 = local read "Pitch 5 (deg)"() -> (w367:dbl)
            n261 = local read "Pitch 6 (deg)"() -> (w369:dbl)
            n262 = local read "Pitch 7 (deg)"() -> (w371:dbl)
            n263 = local read "Pitch 8 (deg)"() -> (w373:dbl)
            n264 = local read "Yaw 1 (deg)"() -> (w358:dbl)
            n265 = local read "Pitch (deg)"() -> (w359:dbl)
            n266 = local read "Yaw 2 (deg)"() -> (w360:dbl)
            n267 = local read "Yaw 4 (deg)"() -> (w364:dbl)
            n268 = local read "Yaw 5 (deg)"() -> (w366:dbl)
            n269 = local read "Yaw 6 (deg)"() -> (w368:dbl)
            n270 = local read "Yaw 7 (deg)"() -> (w370:dbl)
            n271 = local read "Yaw 8 (deg)"() -> (w372:dbl)
            n272 = local read "Yaw 3 (deg)"() -> (w362:dbl)
            n273 = local read "Coil 1"() -> (w407:cluster{"X (m)":sgl, "Y (m)":sgl, "Z (m)":sgl})
            n274 = local read "Coil 2"() -> (w406:cluster{"X (m)":sgl, "Y (m)":sgl, "Z (m)":sgl})
            n275 = local read "Coil 3"() -> (w405:cluster{"X (m)":sgl, "Y (m)":sgl, "Z (m)":sgl})
            n276 = local read "Coil 4"() -> (w404:cluster{"X (m)":sgl, "Y (m)":sgl, "Z (m)":sgl})
            n277 = local read "Coil 5"() -> (w403:cluster{"X (m)":sgl, "Y (m)":sgl, "Z (m)":sgl})
            n278 = local read "Coil 6"() -> (w402:cluster{"X (m)":sgl, "Y (m)":sgl, "Z (m)":sgl})
            n279 = local read "Coil 7"() -> (w401:cluster{"X (m)":sgl, "Y (m)":sgl, "Z (m)":sgl})
            n280 = local read "Coil 8"() -> (w400:cluster{"X (m)":sgl, "Y (m)":sgl, "Z (m)":sgl})
            n281 = Cluster To Array(cluster=w407) -> (array=w399:sgl[])
            n282 = Cluster To Array(cluster=w406) -> (array=w398:sgl[])
            n283 = Cluster To Array(cluster=w405) -> (array=w397:sgl[])
            n284 = Cluster To Array(cluster=w404) -> (array=w396:sgl[])
            n285 = Cluster To Array(cluster=w403) -> (array=w395:sgl[])
            n286 = Cluster To Array(cluster=w402) -> (array=w394:sgl[])
            n287 = Cluster To Array(cluster=w401) -> (array=w393:sgl[])
            n288 = Cluster To Array(cluster=w400) -> (array=w392:sgl[])
            n289 = Build Array(w399, w398, w397, w396, w395, w394, w393, w392) -> (w380:sgl[][])
            n290 = Build Array(w374, w358, w359) -> (w357:dbl[])
            n291 = Build Array(w374, w360, w361) -> (w356:dbl[])
            n292 = Build Array(w374, w362, w363) -> (w355:dbl[])
            n293 = Build Array(w374, w364, w365) -> (w354:dbl[])
            n294 = Build Array(w374, w366, w367) -> (w353:dbl[])
            n295 = Build Array(w374, w368, w369) -> (w352:dbl[])
            n296 = Build Array(w374, w370, w371) -> (w351:dbl[])
            n297 = Build Array(w374, w372, w373) -> (w350:dbl[])
            n298 = Build Array(w357, w356, w355, w354, w353, w352, w351, w350) -> (w349:dbl[][])
            n299 = script code="cd ('C:\\EMTS_SIMU')\nglobal C r \n\n\nPOR=[rs(1) rs(2) rs(3) os(2) os(3) ];\n\n%P_O_Cal_fix;"("??"=w391, "p"=w429, "f"=w428, "o"=w427, "N_sende"=w419, "N_empfang"=w418, "R_sende"=w417, "R_empfang"=w416, "Ia"=w426, "A_Empfang"=w425, "Verstaerkung"=w424, "U"=w347, "r"=w380, "StartX"=w379, "StartY"=w378, "StartZ"=w377, "StartPhi"=w376, "StartTheta"=w375, "oo"=w349) -> ("??"=w390:errorcluster, "POR"=w421:dbl[])
          }
          frame True {
            w585 = 1.0
            n300 = local read "Sensor static ?"() -> (w535:bool)
            n301 = case shown="False" w535 {
              tunnel: [w610 w654] -> w581
              tunnel: [w609 w653] -> w572
              tunnel: [w608 w652] -> w571
              tunnel: [w607 w651] -> w570
              tunnel: [w606 w650] -> w569
              tunnel: [w605 w649] -> w568
              tunnel: [w604 w648] -> w567
              tunnel: [w603 w647] -> w566
              tunnel: [w602 w646] -> w565
              frame False {
                n302 = local read "Sensor coil move"() -> (w611:cluster{"X (m)":sgl, "Y (m)":sgl, "Z (m)":sgl})
                n303 = local read "Coil 1"() -> (w644:cluster{"X (m)":sgl, "Y (m)":sgl, "Z (m)":sgl})
                n304 = local read "Coil 2"() -> (w643:cluster{"X (m)":sgl, "Y (m)":sgl, "Z (m)":sgl})
                n305 = local read "Coil 3"() -> (w642:cluster{"X (m)":sgl, "Y (m)":sgl, "Z (m)":sgl})
                n306 = local read "Coil 4"() -> (w641:cluster{"X (m)":sgl, "Y (m)":sgl, "Z (m)":sgl})
                n307 = local read "Coil 5"() -> (w640:cluster{"X (m)":sgl, "Y (m)":sgl, "Z (m)":sgl})
                n308 = local read "Coil 6"() -> (w639:cluster{"X (m)":sgl, "Y (m)":sgl, "Z (m)":sgl})
                n309 = local read "Coil 7"() -> (w638:cluster{"X (m)":sgl, "Y (m)":sgl, "Z (m)":sgl})
                n310 = local read "Coil 8"() -> (w637:cluster{"X (m)":sgl, "Y (m)":sgl, "Z (m)":sgl})
                n311 = Cluster To Array(cluster=w639) -> (array=w632:sgl[])
                n312 = Cluster To Array(cluster=w638) -> (array=w631:sgl[])
                n313 = Cluster To Array(cluster=w644) -> (array=w620:sgl[])
                n314 = Cluster To Array(cluster=w643) -> (array=w636:sgl[])
                n315 = Cluster To Array(cluster=w642) -> (array=w635:sgl[])
                n316 = Cluster To Array(cluster=w641) -> (array=w634:sgl[])
                n317 = Cluster To Array(cluster=w640) -> (array=w633:sgl[])
                n318 = Cluster To Array(cluster=w637) -> (array=w630:sgl[])
                n319 = Cluster To Array(cluster=w611) -> (array=w629:sgl[])
                n320 = To Double Precision Float(number=w634) -> (double precision float=w625:dbl[])
                n321 = To Double Precision Float(number=w633) -> (double precision float=w624:dbl[])
                n322 = To Double Precision Float(number=w632) -> (double precision float=w623:dbl[])
                n323 = To Double Precision Float(number=w631) -> (double precision float=w622:dbl[])
                n324 = To Double Precision Float(number=w630) -> (double precision float=w621:dbl[])
                n325 = To Double Precision Float(number=w629) -> (double precision float=w602:dbl[])
                n326 = To Double Precision Float(number=w620) -> (double precision float=w628:dbl[])
                n327 = To Double Precision Float(number=w636) -> (double precision float=w627:dbl[])
                n328 = To Double Precision Float(number=w635) -> (double precision float=w626:dbl[])
                n329 = Rotate 1D Array(1:w628, 2:0 ("n")) -> (0:w610:dbl[])
                n330 = Rotate 1D Array(1:w627, 2:0 ("n")) -> (0:w609:dbl[])
                n331 = Rotate 1D Array(1:w626, 2:0 ("n")) -> (0:w608:dbl[])
                n332 = Rotate 1D Array(1:w625, 2:0 ("n")) -> (0:w607:dbl[])
                n333 = Rotate 1D Array(1:w624, 2:0 ("n")) -> (0:w606:dbl[])
                n334 = Rotate 1D Array(1:w623, 2:0 ("n")) -> (0:w605:dbl[])
                n335 = Rotate 1D Array(1:w622, 2:0 ("n")) -> (0:w604:dbl[])
                n336 = Rotate 1D Array(1:w621, 2:0 ("n")) -> (0:w603:dbl[])
              }
              frame True {
                n337 = local read "Coil 1"() -> (w671:cluster{"X (m)":sgl, "Y (m)":sgl, "Z (m)":sgl})
                n338 = local read "Coil 2"() -> (w670:cluster{"X (m)":sgl, "Y (m)":sgl, "Z (m)":sgl})
                n339 = local read "Coil 3"() -> (w669:cluster{"X (m)":sgl, "Y (m)":sgl, "Z (m)":sgl})
                n340 = local read "Coil 4"() -> (w668:cluster{"X (m)":sgl, "Y (m)":sgl, "Z (m)":sgl})
                n341 = local read "Coil 5"() -> (w667:cluster{"X (m)":sgl, "Y (m)":sgl, "Z (m)":sgl})
                n342 = local read "Coil 6"() -> (w666:cluster{"X (m)":sgl, "Y (m)":sgl, "Z (m)":sgl})
                n343 = local read "Coil 7"() -> (w665:cluster{"X (m)":sgl, "Y (m)":sgl, "Z (m)":sgl})
                n344 = local read "Coil 8"() -> (w664:cluster{"X (m)":sgl, "Y (m)":sgl, "Z (m)":sgl})
                n345 = local read "Sensor coil"() -> (w663:cluster{"X (m)":sgl, "Y (m)":sgl, "Z (m)":sgl})
                n346 = Cluster To Array(cluster=w666) -> (array=w658:sgl[])
                n347 = Cluster To Array(cluster=w665) -> (array=w657:sgl[])
                n348 = Cluster To Array(cluster=w671) -> (array=w645:sgl[])
                n349 = Cluster To Array(cluster=w670) -> (array=w662:sgl[])
                n350 = Cluster To Array(cluster=w669) -> (array=w661:sgl[])
                n351 = Cluster To Array(cluster=w668) -> (array=w660:sgl[])
                n352 = Cluster To Array(cluster=w667) -> (array=w659:sgl[])
                n353 = Cluster To Array(cluster=w664) -> (array=w656:sgl[])
                n354 = Cluster To Array(cluster=w663) -> (array=w655:sgl[])
                n355 = To Double Precision Float(number=w645) -> (double precision float=w654:dbl[])
                n356 = To Double Precision Float(number=w662) -> (double precision float=w653:dbl[])
                n357 = To Double Precision Float(number=w661) -> (double precision float=w652:dbl[])
                n358 = To Double Precision Float(number=w660) -> (double precision float=w651:dbl[])
                n359 = To Double Precision Float(number=w659) -> (double precision float=w650:dbl[])
                n360 = To Double Precision Float(number=w658) -> (double precision float=w649:dbl[])
                n361 = To Double Precision Float(number=w657) -> (double precision float=w648:dbl[])
                n362 = To Double Precision Float(number=w656) -> (double precision float=w647:dbl[])
                n363 = To Double Precision Float(number=w655) -> (double precision float=w646:dbl[])
              }
            }
            n364 = local read "Noise Level (dBW)"() -> (w543:dbl)
            n365 = local read "Pitch 3 (deg)"() -> (w596:dbl)
            n366 = local read "Pitch (deg)"() -> (w583:dbl)
            n367 = local read "Pitch 2 (deg)"() -> (w598:dbl)
            n368 = local read "Pitch 4 (deg)"() -> (w594:dbl)
            n369 = local read "Pitch 5 (deg)"() -> (w592:dbl)
            n370 = local read "Pitch 6 (deg)"() -> (w590:dbl)
            n371 = local read "Pitch 7 (deg)"() -> (w588:dbl)
            n372 = local read "Pitch 8 (deg)"() -> (w586:dbl)
            n373 = local read "Noise On ?"() -> (w541:bool)
            n374 = local read "Yaw 1 (deg)"() -> (w601:dbl)
            n375 = local read "Pitch (deg)"() -> (w600:dbl)
            n376 = local read "Yaw 2 (deg)"() -> (w599:dbl)
            n377 = local read "Yaw 4 (deg)"() -> (w595:dbl)
            n378 = local read "Yaw 5 (deg)"() -> (w593:dbl)
            n379 = local read "Yaw 6 (deg)"() -> (w591:dbl)
            n380 = local read "Yaw 7 (deg)"() -> (w589:dbl)
            n381 = local read "Yaw 8 (deg)"() -> (w587:dbl)
            n382 = local read "Yaw 3 (deg)"() -> (w597:dbl)
            n383 = local read "Yaw (deg)"() -> (w584:dbl)
            n384 = case shown="False" w541 {
              tunnel: [-inf w673] -> w542
              tunnel: w543 -> [_ w673]
              frame False {
              }
              frame True {
              }
            }
            n385 = Build Array(w585, w601, w600) -> (w582:dbl[])
            n386 = Build Array(w585, w599, w598) -> (w580:dbl[])
            n387 = Build Array(w585, w597, w596) -> (w579:dbl[])
            n388 = Build Array(w585, w595, w594) -> (w578:dbl[])
            n389 = Build Array(w585, w593, w592) -> (w577:dbl[])
            n390 = Build Array(w585, w591, w590) -> (w576:dbl[])
            n391 = Build Array(w585, w589, w588) -> (w575:dbl[])
            n392 = Build Array(w585, w587, w586) -> (w574:dbl[])
            n393 = Build Array(w585, w584, w583) -> (w573:dbl[])
            n394 = script code="cd ('C:\\EMTS_SIMU')\ns=n_sample;\n%noise=wgn(1,s,nl);\n\nB_U_Cal_fix_2;"("??"=w532, "r1"=w581, "r2"=w572, "r3"=w571, "r4"=w570, "r5"=w569, "r6"=w568, "r7"=w567, "r8"=w566, "rs"=w565, "o1"=w582, "o2"=w580, "o3"=w579, "o4"=w578, "o5"=w577, "o6"=w576, "o7"=w575, "o8"=w574, "os"=w573, "N_sende"=w559, "L"=w563, "N_empfang"=w558, "R_sende"=w557, "R_empfang"=w556, "Ug"=w544, "f"=w564, "nl"=w542, "n_sample"=w547, "delta_t"=w546, "flag"=w545) -> ("??"=w549:errorcluster, "rs"=w562:dbl[], "f"=w561:dbl, "os"=w560:dbl[], "Ia"=w555:dbl, "A_Empfang"=w554:dbl, "Verstaerkung"=w553:dbl, "U1"=w533:dbl[], "r"=w550:dbl[][], "oo"=w552:dbl[][], "V_Visual"=w540:dbl[][], "U_norm"=w531:dbl[])
            n395 = script code="cd ('C:\\EMTS_SIMU')\nglobal C r \n\nPOR=[rs(1) rs(2) rs(3) os(2) os(3) ];\n\n%P_O_Cal_fix;"("??"=w549, "p"=w562, "f"=w561, "o"=w560, "N_sende"=w559, "N_empfang"=w558, "R_sende"=w557, "R_empfang"=w556, "Ia"=w555, "A_Empfang"=w554, "Verstaerkung"=w553, "U"=w531, "r"=w550, "oo"=w552, "StartX"=w534, "StartY"=w539, "StartZ"=w538, "StartPhi"=w537, "StartTheta"=w536) -> ("??"=w548:errorcluster, "POR"=w551:dbl[])
          }
        }
        "Real sensor's P&O" <- w343
        "Measured Voltage" <- w328
        "Simulated voltage induced by each transmitter coil (V)" <- w345
        "U_norm" <- w322
        n396 = local read "stop"() -> (w344:bool)
        n397 = Wait (ms)(milliseconds to wait=u32 5) -> ()  [unwired: 1 out]
        n398 = disable-structure shown="Disabled" {
          disable-tunnel: _ -> [w674 _]
          frame Disabled {
            "Estimated sensor's P&O" <- w674
          }
          frame Enabled {
          }
        }
      }
    }
  }
  n399 = while {
    stop <- w686 stop-if-true
    n400 = case shown="0, Default" "Select Waveform" {
      tunnel: ["a*sin(w*t)" ("formula") w693 w699] -> w681
      tunnel: ["Sine Frequency (Hz)" w692 w698] -> w680
      tunnel: [w688 w697 w704] -> w675
      tunnel: ["Sampling info (sine)" "Sampling info (ramp)" "Sampling info (DC)"] -> w678
      tunnel: [w687 w695 w702] -> w676
      frame 0, Default {
        n401 = Unbundle By Name("Sampling info (sine)") -> ("#s"=w688:dbl, "Fs"=w687:dbl)
        "Signal Frequency" <- "Sine Frequency (Hz)"
      }
      frame 1 {
        w692 = 100.0
        n402 = local write "Signal Frequency"(w692) -> ()
        n403 = call "RampFomular (SubVI).vi"("Ramp Voltage (V)"="Ramp Voltage (V)", "num"=w692) -> ("concatenated string"=w693:string)  [unwired: 8 in, 1 out]
        "concatenated string" <- w693
        n404 = Unbundle By Name("Sampling info (ramp)") -> ("#s"=w697:dbl, "Fs"=w695:dbl)
      }
      frame 2 {
        w698 = 100.0
        n405 = local write "Signal Frequency"(w698) -> ()
        n406 = To Quad Integer(1:"DC  (V)") -> (0:w701:i64)
        n407 = Unbundle By Name("Sampling info (DC)") -> ("#s"=w704:dbl, "Fs"=w702:dbl)
        n408 = Number To Decimal String(number=w701) -> (decimal integer string=w699:string)  [unwired: 1 in]
      }
    }
    "#s" <- w675
    n409 = Divide(x=w675, y=w676) -> (x/y=→"delta_t":dbl)
    n410 = call <vilib>:"Formula Waveform.vi"("sampling info"=w678, "reset signal"="Reset Signal", "formula"=w681, "amplitude"="Sine Voltage (V)", "frequency"=w680) -> ("signal out"=→"Signal Generation":waveform(dbl))  [unwired: 5 in, 1 out]
    n411 = local read "stop"() -> (w686:bool)
    n412 = Wait (ms)(milliseconds to wait=u32 5) -> ()  [unwired: 1 out]
  }
  n413 = disable-structure shown="Disabled" {
    frame Disabled {
      n414 = flat-sequence {
        frame #0 {
          n415 = Wait (ms)(milliseconds to wait=u32 2000 ("millisecond timer value")) -> ()  [unwired: 1 out]
        }
        frame #1 {
          n416 = for {
            N: 100 -> [_]
            i -> [w707]
            n417 = flat-sequence {
              frame #0 {
                n418 = local read "Simulated voltage induced by each transmitter coil (V)"() -> (w708:dbl[])
                n419 = local read "Real sensor's P&O"() -> (w712:dbl[])
                n420 = local read "U_norm"() -> (w719:dbl[])
                n421 = call-poly <vilib>:"Write To Spreadsheet File.vi"("format (%.3f)"="%.8f", "append to file? (new file:F)"=TRUE, "1D data"=w719, "file path (dialog if empty)"=path "d:/0630/Um_Noise") -> ()  [unwired: 4 in, 1 out]
                n422 = call-poly <vilib>:"Write To Spreadsheet File.vi"("format (%.3f)"="%.8f", "append to file? (new file:F)"=TRUE, "1D data"=w712, "file path (dialog if empty)"=path "d:/0630/POR") -> ()  [unwired: 4 in, 1 out]
                n423 = call-poly <vilib>:"Write To Spreadsheet File.vi"("format (%.3f)"="%.8f", "append to file? (new file:F)"=TRUE, "1D data"=w708, "file path (dialog if empty)"=path "d:/0630/Um_NoNoise") -> ()  [unwired: 4 in, 1 out]
              }
              frame #1 {
                n424 = Wait (ms)(milliseconds to wait=u32 1000) -> ()  [unwired: 1 out]
              }
            }
            "Times" <- w707
          }
        }
      }
    }
    frame Enabled {
    }
  }
  n425 = call <vilib>:"Simple Error Handler.vi"("type of dialog (OK msg:1)"=w7, "error in (no error)"=w6) -> ()  [unwired: 3 in, 5 out]
  n426 = Divide(x=w4, y=u32 1000) -> (x/y=→"Time needed (s)":dbl)
